vi "Find Engine from Child.vi"(8 "error in (no error)":errorcluster, 10 "Node ID":string, 11 "HW Engine":refnum<data-value>) -> (0 "error out":errorcluster, 3 "Engine":refnum<data-value>)   [LabVIEW 2025, in "Config Tool.lvlib"]
uses:
  Config Tool.lvlib
  Users/Public/Documents/Sandia National Labs/TSS Plugin/CEF.lvlibp/Node/CEF_Node.lvclass
  <vilib>/Utility/error.llb/Trim Whitespace One-Sided.vi
  Users/Public/Documents/Sandia National Labs/TSS Plugin/CEF.lvlibp/Node/ReadChildren.vi
  Users/Public/Documents/Sandia National Labs/TSS Plugin/CEF.lvlibp/Node/ReadParent.vi
  Users/Public/Documents/Sandia National Labs/TSS Plugin/CEF.lvlibp
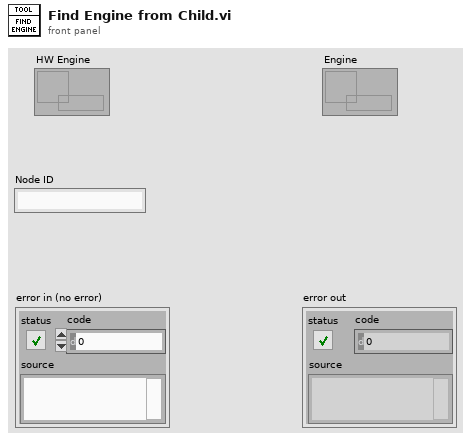
[diagram p1: front panel]
types:
  T1 = cluster{"ID":string, "parent ID":string, "node type":string, "text":string, "additional text":string, "glyph":string, "depth":i32, "glyph overlay":string}[]
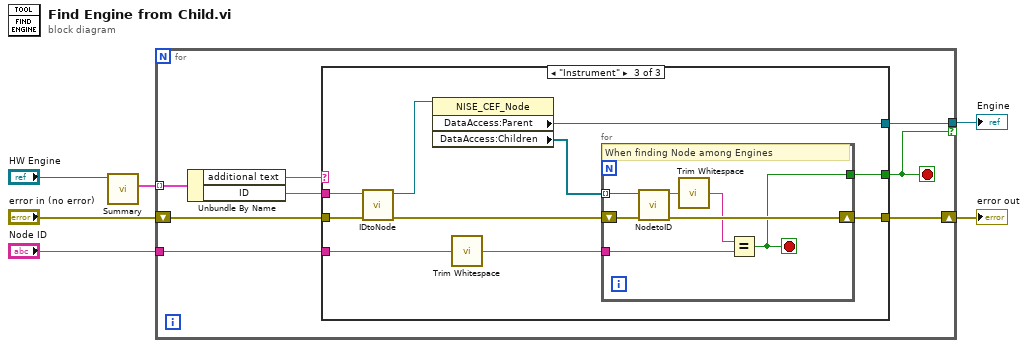
[diagram p0: block diagram]
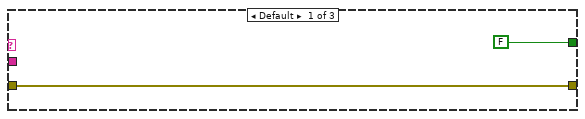
[diagram p2: hidden frame]
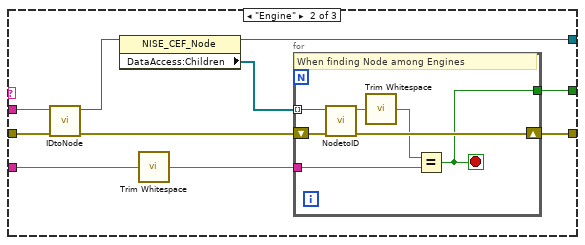
[diagram p3: hidden frame]
diagram:
  n1 = call "Summary.vi"("node self ref"="HW Engine") -> ("summary"=w6:T1)  [unwired: 9 in, 1 out]
  n2 = for {
    tunnel: "Node ID" -> [w13]
    tunnel: w6 -> [w14] mode=indexing
    shift-right: [w10] -> w2
    shift-left: "error in (no error)" -> [w11]
    tunnel: [w9] -> w1 if=w8
    stop <- w8 stop-if-true
    n3 = Unbundle By Name(w14) -> ("additional text"=w7:string, "ID"=w12:string)
    n4 = case shown="\"Instrument\"" w7 {
      tunnel: w13 -> [_ w23 w41]
      tunnel: w12 -> [_ w21 w39]
      tunnel: w11 -> [w16 w26 w43]
      tunnel: [w16 w22 w40] -> w10
      tunnel: [FALSE w20 w38] -> w8
      tunnel: [_ w19 w34] -> w9
      frame Default {
      }
      frame "Engine" {
        n5 = call "IDtoNode.vi"("error in"=w26, "ID"=w21) -> ("error out"=w17:errorcluster, "node ref"=w25:refnum<data-value>)  [unwired: 7 in, 1 out]
        n6 = property class="NISE_CEF_Node"(reference=w25) -> (reference out=w19:refnum<data-value>, "DataAccess:Children"=w24:refnum<data-value>[])  [unwired: 1 in, 1 out]
        n7 = call <vilib>:"Trim Whitespace.vi"("string"=w23) -> ("trimmed string"=w18:string)  [unwired: 1 in]
        n8 = for {
          tunnel: w24 -> [w33] mode=indexing
          tunnel: w18 -> [w32]
          shift-right: [w30] -> w22
          shift-left: w17 -> [w31]
          tunnel: [w28] -> w20
          stop <- w28 stop-if-true
          # "When finding Node among Engines"
          n9 = call "NodetoID.vi"("error in"=w31, "node ref"=w33) -> ("error out"=w30:errorcluster, "ID"=w29:string)  [unwired: 8 in]
          n10 = call <vilib>:"Trim Whitespace.vi"("string"=w29) -> ("trimmed string"=w27:string)  [unwired: 1 in]
          n11 = Equal?(x=w27, y=w32) -> (x = y?=w28:bool)
        }
      }
      frame "Instrument" {
        n12 = call "IDtoNode.vi"("error in"=w43, "ID"=w39) -> ("error out"=w36:errorcluster, "node ref"=w42:refnum<data-value>)  [unwired: 7 in, 1 out]
        n13 = property class="NISE_CEF_Node"(reference=w42) -> ("DataAccess:Parent"=w34:refnum<data-value>, "DataAccess:Children"=w35:refnum<data-value>[])  [unwired: 1 in, 2 out]
        n14 = call <vilib>:"Trim Whitespace.vi"("string"=w41) -> ("trimmed string"=w37:string)  [unwired: 1 in]
        n15 = for {
          tunnel: w35 -> [w50] mode=indexing
          tunnel: w37 -> [w49]
          shift-right: [w47] -> w40
          shift-left: w36 -> [w48]
          tunnel: [w45] -> w38
          stop <- w45 stop-if-true
          # "When finding Node among Engines"
          n16 = call "NodetoID.vi"("error in"=w48, "node ref"=w50) -> ("error out"=w47:errorcluster, "ID"=w46:string)  [unwired: 8 in]
          n17 = call <vilib>:"Trim Whitespace.vi"("string"=w46) -> ("trimmed string"=w44:string)  [unwired: 1 in]
          n18 = Equal?(x=w44, y=w49) -> (x = y?=w45:bool)
        }
      }
    }
  }
  "error out" <- w2
  "Engine" <- w1
